vi "_Agilent DMM Tree.vi"   [LabVIEW 2011]
uses:
  DMM Command.ctl
panel:
  # "See Diagram"
types:
  T1 = typedef "DMM Command.ctl" = enum16{"LOAD", "INITIALIZE", "PRESET", "GET STIMULUS", "SET STIMULUS", "MEASURE", "RELEASE", "UNLOAD", "GET CALIBRATION", "CALIBRATE"}
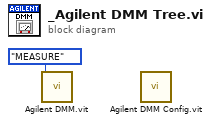
[diagram p0: block diagram]
diagram:
  n1 = call "Agilent DMM.vit"("DMM Command"=DMM_Command."MEASURE" ("VNA Command")) -> ()  [unwired: 4 in, 7 out]
  n2 = call "Agilent DMM Config.vit"() -> ()  [unwired: 2 in, 10 out]
